vi "clear_com.vi"() -> ()   [LabVIEW 2011]
panel:
  in  "VISA session":refnum<visa-resource-name>
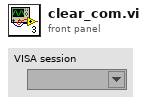
[diagram p1: front panel]
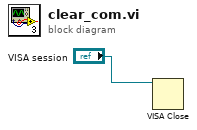
[diagram p0: block diagram]
diagram:
  n1 = VISA Close(VISA resource name="VISA session") -> ()  [unwired: 1 in, 1 out]
